vi "CalcTheta.vi"() -> (3 "ThetaValues":dbl[](array[numeric]))   [LabVIEW 2019]
panel:
  # "Front of bot"
  # "L"
  # "W"
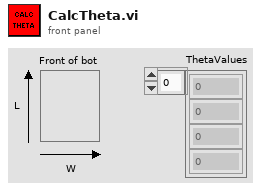
[diagram p1: front panel]
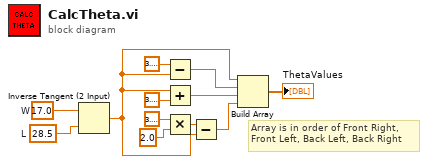
[diagram p0: block diagram]
diagram:
  w10 = 17.0  # W
  w9 = 28.5  # L
  # "Array is in order of Front Right,\nFront Left, Back Left, Back Right"
  n1 = Inverse Tangent (2 Input)(1:w9, 2:w10) -> (0:w1:dbl)
  n2 = Subtract(x=3.141592653589793, y=w1) -> (x-y=w2:dbl)
  n3 = Add(x=w1, y=3.141592653589793) -> (x+y=w4:dbl)
  n4 = Multiply(x=3.141592653589793, y=2.0) -> (x*y=w6:dbl)
  n5 = Subtract(x=w6, y=w1) -> (x-y=w5:dbl)
  n6 = Build Array(w1, w2, w4, w5) -> (→"ThetaValues":dbl[])
